vi "V2 Measurement Service Constant.vi"() -> (3 "provided_interface":string)   [LabVIEW 2021, in "MeasurementClient Editor.lvlib"]
uses:
  MeasurementClient Editor.lvlib
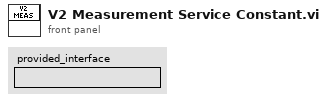
[diagram p1: front panel]
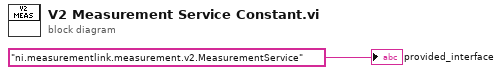
[diagram p0: block diagram]
diagram:
  "provided_interface" <- "ni.measurementlink.measurement.v2.MeasurementService" ("provided_interface")
